vi "Winding.vi"(8 "Error In":errorcluster, 11 "AutoData":T1) -> (0 "Error Out":errorcluster, 3 "AutoData out":T1)   [LabVIEW 2019, in "AutoMode.lvlib"]
uses:
  AutoMode.lvlib
  Cluster - AutoModeData.ctl
  MainController/Cluster - TestSettings.ctl
  MainController/Cluster - HardwareConfiguration.ctl
  MainController/Cluster - TestResults.ctl
  Cluster - AutoModeMessage.ctl
  Enum - AutoModeState.ctl
  MainController/Cluster - MainControllerMessage.ctl
  MainController/Enum - MainState.ctl
  Mark10 API/WriteSpeed.vi
  Mark10 API/WriteCCWTravelLimit.vi
  Mark10 API/WriteMoveCrossheadCCW.vi
  Mark10 API/Mark 10 TSTM-DC.lvlib
  Timer/Timer.lvlib
  EventLogger/EventLogger.lvlib
  MainController/MainController.lvlib
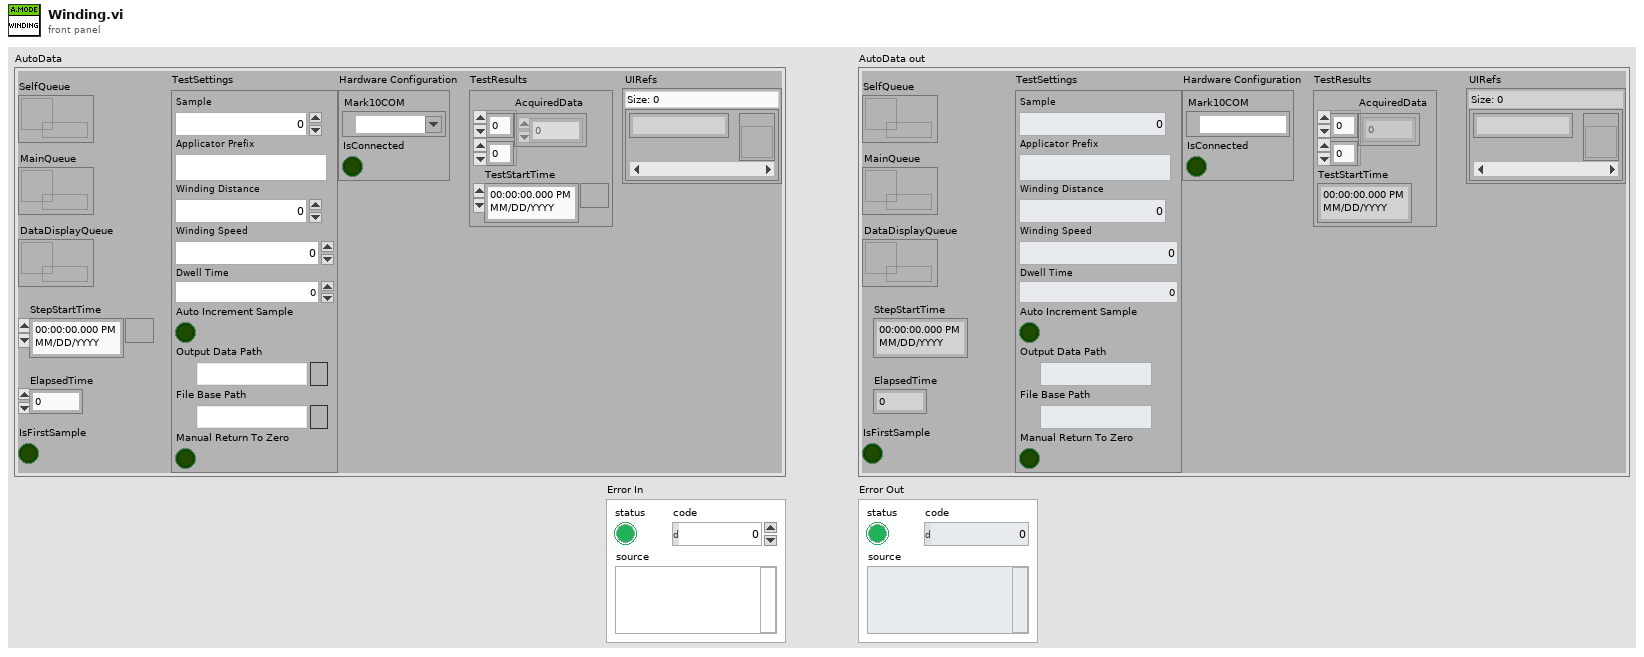
[diagram p1: front panel]
types:
  T1 = typedef "AutoMode.lvlib/Cluster - AutoModeData.ctl" = cluster{"DataDisplayQueue":refnum<queue>, "StepStartTime":timestamp, "TestSettings":T2, "Hardware Configuration":T3, "TestResults":T4, "ElapsedTime":dbl, "IsFirstSample":bool, "SelfQueue":refnum<queue>, "MainQueue":refnum<queue>, "UIRefs":map{string, refnum<vi>}}
  T2 = typedef "MainController.lvlib/Cluster - TestSettings.ctl" = cluster{"Sample":u32, "Applicator Prefix":string, "Winding Distance":dbl, "Winding Speed":dbl, "Dwell Time":dbl, "Auto Increment Sample":bool, "Output Data Path":path, "File Base Path":path, "Manual Return To Zero":bool}
  T3 = typedef "MainController.lvlib/Cluster - HardwareConfiguration.ctl" = cluster{"Mark10COM":refnum<visa-resource-name>, "IsConnected":bool}
  T4 = typedef "MainController.lvlib/Cluster - TestResults.ctl" = cluster{"AcquiredData":dbl[][], "TestStartTime":timestamp}
  T5 = typedef "AutoMode.lvlib/Enum - AutoModeState.ctl" = enum16{"Initialize", "Idle", "UpdateConfig", "UpdateHWConfig", "BroadcastSettings", "Start", "CheckValidReportPath", "Winding", "WaitForWinding", "Unwind", "WaitForUnwind", "Stop", "Abort", "WriteDataToFile", "EventTriggered", "GenerateFilePath", "ZeroPosition", "GotoZero", "Error", "Exit"}
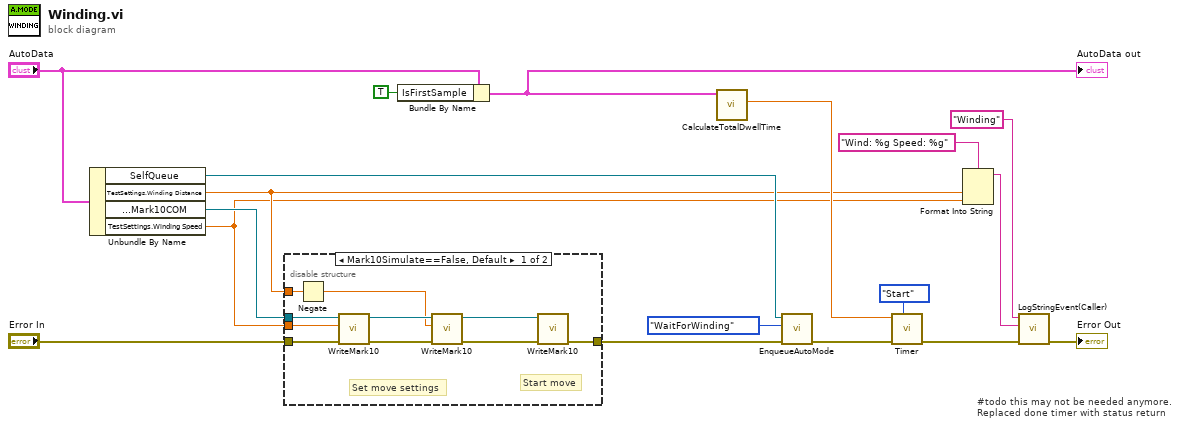
[diagram p0: block diagram]
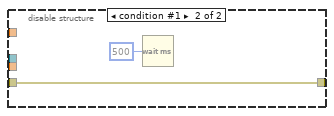
[diagram p2: hidden frame]
diagram:
  # "#todo this may not be needed anymore.\nReplaced done timer with status return"
  n1 = Unbundle By Name("AutoData") -> ("SelfQueue"=w7:refnum<queue>, "TestSettings.Winding Distance"=w3:dbl, "Hardware Configuration.Mark10COM"=w18:refnum<visa-resource-name>, "TestSettings.Winding Speed"=w2:dbl)
  n2 = disable-structure shown="Mark10Simulate==False, Default" {
    disable-tunnel: w3 -> [w27 _]
    disable-tunnel: w2 -> [w26 _]
    disable-tunnel: w18 -> [w25 _]
    disable-tunnel: "Error In" -> [w20 w30]
    disable-tunnel: [w19 w30] -> w15
    frame condition #0 (active) {
      # "Start move"
      # "Set move settings"
      n3 = Negate(x=w27) -> (-x=w21:dbl)
      n4 = call-poly "WriteMark10.vi"("error in"=w20, "Speed"=w26, "VISA resource name"=w25) -> ("error out"=w24:errorcluster, "VISA resource name out"=w28:refnum<visa-resource-name>)  [unwired: 7 in]
      n5 = call-poly "WriteMark10.vi"("error in"=w24, "CCWTravelLimit"=w21, "VISA resource name"=w28) -> ("error out"=w22:errorcluster, "VISA resource name out"=w23:refnum<visa-resource-name>)  [unwired: 7 in]
      n6 = call-poly "WriteMark10.vi"("error in"=w22, "VISA resource name"=w23) -> ("error out"=w19:errorcluster)  [unwired: 8 in, 1 out]
    }
    frame condition #1 {
      n7 = Wait (ms)(milliseconds to wait=u32 500) -> ()  [unwired: 1 out]
    }
  }
  n8 = Bundle By Name(cluster="AutoData", "IsFirstSample"=TRUE) -> (w8:T1)
  "AutoData out" <- w8
  n9 = call "CalculateTotalDwellTime.vi"("AutoData"=w8) -> ("DwellTime"=w14:dbl)  [unwired: 10 in]
  n10 = call "EnqueueAutoMode.vi"("error in (no error)"=w15, "AutoState"=Enum_-_AutoModeState."WaitForWinding" ("CycleTestState"), "Queue in"=w7) -> ("error out"=w17:errorcluster)  [unwired: 7 in, 1 out]
  n11 = call "Timer.vi"("TimerState"=enum16{"Reset", "Start", "GetTime", "Stop"}."Start", "Error In"=w17, "TargetTime(ms)"=w14) -> ("Error Out"=w11:errorcluster)  [unwired: 7 in, 1 out]
  n12 = Format Into String(format string="Wind: %g Speed: %g", w3, w2) -> (resulting string=w1:string)  [unwired: 2 in, 1 out]
  n13 = call "LogStringEvent(Caller).vi"("Error In"=w11, "Data"=w1, "Field"="Winding") -> ("Error Out"=→"Error Out":errorcluster)  [unwired: 8 in]
